vi "Send message to Top.vi"(6 "Error in (no error)":errorcluster, 8 "Data":variant, 9 "Response":string, 10 "Module":T2, 11 "Mailbox address in":T1) -> (0 "Error out":errorcluster, 3 "Mailbox address out":T1)   [LabVIEW 2021]
doc: "Sends message cluster as [variant] which compose of:\nModule [enum]- name of module who sends message. To recognise origin of message.\nResponse [string]- name of response.\nData [variant]- any type of data that has to be send.\nTime [timestamp]- time when message was send.\n\nNote: If there is an error on the input, word \"Error\" is concated before Response and Data are replaced by error cluster."
uses:
  Data types/Module name.ctl
  Data types/Mailbox address.ctl
  Data types/MSG to TOP.ctl
  MessengerLib.lvlib
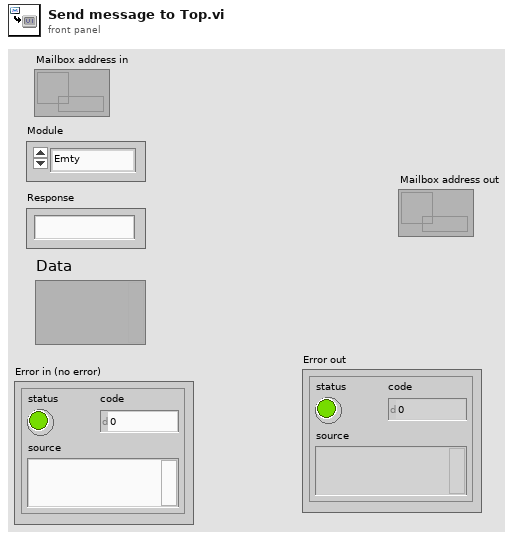
[diagram p1: front panel]
types:
  T1 = typedef "MessengerLib.lvlib/Mailbox address.ctl" = refnum<queue>
  T2 = typedef "MessengerLib.lvlib/Module name.ctl" = enum16{"Emty", "Magnet", "VTI", "Excitation", "Servo", "Acquisition", "Rotator", "Digitizer", "SMU2450", "Carousel", "Multimeter", "Tmp monitor", "Power monitor"}
  T3 = typedef "MessengerLib.lvlib/MSG to TOP.ctl" = cluster{"Module":T2, "Response":string, "Data":variant, "Time":timestamp}
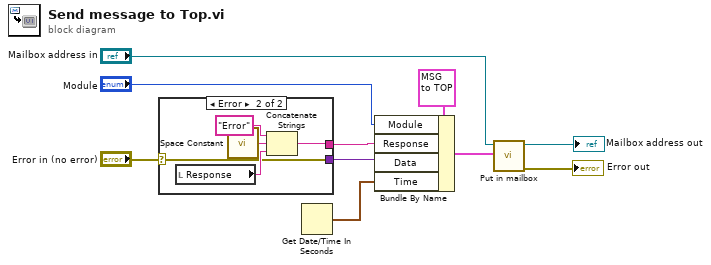
[diagram p0: block diagram]
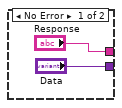
[diagram p2: hidden frame]
diagram:
  n1 = case shown="Error" "Error in (no error)" {
    selector: "Error in (no error)" -> [_ w13]
    tunnel: ["Data" w13] -> w7
    tunnel: ["Response" w14] -> w6
    frame No Error {
    }
    frame Error {
      n2 = local read "Response"() -> (w15:string)
      n3 = call <vilib>:"Space Constant.vi"() -> ("String"=w17:string)
      n4 = Concatenate Strings("Error" ("Response"), w17, w15) -> (w14:string)
    }
  }
  n5 = Get Date/Time In Seconds() -> (seconds since 1Jan1904=w10:timestamp)
  n6 = Bundle By Name(cluster=T3 {"Module"=enum."Emty", "Response"="", "Data"=variant, "Time"=timestamp(0 s since 1904-01-01)} ("MSG to UI"), "Module"="Module", "Response"=w6, "Data"=w7, "Time"=w10) -> (w5:T3)
  n7 = call "Put in mailbox.vi"("Message"=w5, "Queue in"="Mailbox address in") -> ("error out"=→"Error out":errorcluster, "Queue out"=→"Mailbox address out":refnum<queue>)  [unwired: 7 in, 1 out]
